vi "Controller Test Bench (14).vi"() -> ()   [LabVIEW 2022 SP3]
uses:
  WhiteNoise.ctl
  <vilib>/addons/System Identification/Model Typedefs.llb/si_generic model.ctl
  <vilib>/addons/System Identification/Model Typedefs.llb/SI Model Type.ctl
  <vilib>/addons/System Identification/Model Typedefs.llb/si_variables.ctl
  <vilib>/sound2/lvsound2.llb/Sound Data Format.ctl
  <vilib>/Utility/error.llb/DialogType.ctl
  <vilib>/sound2/lvsound2.llb/Sampling Mode.ctl
  <vilib>/Platform/TimedLoop/XDataNode/timing_clust.ctl
  <vilib>/Platform/TimedLoop/XDataNode/nitl_modes.ctl
  <vilib>/Platform/TimedLoop/XDataNode/wakeup.ctl
  <vilib>/Analysis/4window.llb/windowTd.ctl
  <vilib>/sound2/lvsound2.llb/Sound Output Task ID.ctl
  <vilib>/DAQmx/write.llb/DAQmx Write (Analog Wfm 1Chan NSamp).vi
  <vilib>/DAQmx/read.llb/DAQmx Read (Analog 1D Wfm NChan NSamp).vi
  <vilib>/DAQmx/create/channels.llb/DAQmx Create Channel (AI-Acceleration-Accelerometer).vi
  <vilib>/DAQmx/create/channels.llb/DAQmx Create Channel (AO-Voltage-Basic).vi
  <vilib>/DAQmx/configure/timing.llb/DAQmx Timing (Sample Clock).vi
  <vilib>/Platform/TimedLoop/scheduler/LVUserAPI/_suppVIs/Create_1kHz_TSource.vi
  <vilib>/DAQmx/miscellaneous.llb/DAQmx Fill In Error Info.vi
  <vilib>/DAQmx/configure/task.llb/DAQmx Configure Logging (TDMS).vi
  <vilib>/measure/maspectr.llb/FFT Spectrum (Mag-Phase) for N Chan.vi
  <vilib>/sound2/lvsound2.llb/Sound Output Set Volume (Single).vi
  <vilib>/sound2/lvsound2.llb/Sound Output Write (DBL).vi
  <vilib>/addons/control/pid/pid.llb/PID (DBL Array).vi
  <vilib>/sound2/lvsound2.llb/Sound Output Write (DBL Single).vi
  <vilib>/addons/System Identification/Data Preprocess.llb/SI Lowpass Filter (SISO Waveform).vi
  <vilib>/addons/System Identification/Parametric Estimation.llb/SI Estimate Discrete Transfer Function Model (Joint SISO Waveform).vi
  <vilib>/platform/TimedLoop/XDataNode/XDataNode.xnode
  <vilib>/measure/NI_MAPro.lvlib
  <resource>/objmgr/daqmx.rc
  <vilib>/Analysis/NI_AALPro.lvlib
  <vilib>/measure/NI_MABase.lvlib
  <vilib>/Platform/TimedLoop/XDataNode/XDNodeRunTimeDep.lvlib
  <vilib>/addons/control/pid/NI_PID_pid.lvlib
  <vilib>/addons/System Identification/NI_SysID.lvlib
panel:
  out "system model out":T1={"attributes"={"version"="1.0", "model type"=0, "input names"=[], "output names"=[], "notes"=""}, "coefficients"={"A "=[], "B"=[], "F"=[], "C"=[], "D"=[]}, "std deviations"={"A "=[], "B"=[], "F"=[], "C"=[], "D"=[]}, "coefficients covariance"=[], "noise variance"=[], "fs"=0.0, "system info"={"number of inputs"=0, "number of outputs"=0, "A order"=[], "B order"=[], "F order"=[], "C order"=[], "D order"=[], "Delays"=[]}, "kalman gain"=[], "initial state"=[], "trans func"=[], "zeros-poles"=[], "std of trans func"=[], "std of zeros-poles"=[], "trans func (noise)"=[], "std of trans func (noise)"=[], "zeros-poles (noise)"=[], "std of zeros-poles (noise)"=[], "Symbolic State Space Model"={"Symbolic A"=[], "Symbolic B"=[], "Symbolic C"=[], "Symbolic D"=[], "Symbolic K"=[], "Symbolic Initial State"=[]}, "delay"=[], "variables"=[], "grey trans func spec"={"orders of TF model"={" num order"=1, "den order"=2}, "# of zeros/poles at origin"={"zeros/poles"=1, "number "=0}, "delay initial?"=FALSE, "gain initial?"=FALSE}} {"grey trans func spec"."# of zeros/poles at origin"."zeros/poles" items=["zeros", "poles"]; "std of zeros-poles (noise)"."gain" format="%.2f"; "std of zeros-poles (noise)"."poles" format="%.2f"; "std of zeros-poles (noise)"."zeros" format="%.2f"; "zeros-poles (noise)"."gain" format="%.2f"; "zeros-poles (noise)"."poles" format="%.2f"; "zeros-poles (noise)"."zeros" format="%.2f"; "std of trans func (noise)"."alphas" format="%.2f"; "std of trans func (noise)"."betas" format="%.2f"; "trans func (noise)"."alphas" format="%.2f"; "trans func (noise)"."betas" format="%.2f"; "std of zeros-poles"."gain" format="%.2f"; "std of zeros-poles"."poles" format="%.2f"; "std of zeros-poles"."zeros" format="%.2f"; "std of trans func"."alphas" format="%.2f"; "std of trans func"."betas" format="%.2f"; "zeros-poles"."gain" format="%.2f"; "zeros-poles"."poles" format="%.2f"; "zeros-poles"."zeros" format="%.2f"; "trans func"."alphas" format="%.2f"; "trans func"."betas" format="%.2f"; "fs" format="%.2f"; "std deviations"."A" format="%.2f"; "std deviations"."D" format="%.2f"; "std deviations"."C" format="%.2f"; "std deviations"."F" format="%.2f"; "std deviations"."B" format="%.2f"; "coefficients"."A" format="%.2f"; "coefficients"."D" format="%.2f"; "coefficients"."C" format="%.2f"; "coefficients"."F" format="%.2f"; "coefficients"."B" format="%.2f"; "attributes"."model type" items=["Undefined", "AR", "ARX (SISO)", "ARX (MISO)", "ARX (MIMO)", "ARMAX (SISO)", "ARMAX (MISO)", "Output-Error (SISO)", "Output-Error (MISO)", "Box-Jenkins (SISO)", "Box-Jenkins (MISO)", "General Linear (SISO)", "General Linear (MISO)", "State-Space (SISO)", "State-Space (MISO)", "State-Space (MIMO)", "Transfer Function (SISO)", "Transfer Function (MISO)", "Transfer Function (MIMO)", "Zero-Pole-Gain (SISO)", "Zero-Pole-Gain (MISO)", "Zero-Pole-Gain (MIMO)"]}
  out "model coefficients":T4
  out "noise":dbl[](array[numeric])
  in  "Sample Rate":dbl=16384.0
  in  "TimeOut":dbl=30.0 format="%#_13g"
  in  "Cluster":T6={"Seed"=0.0, "Standard Deviation"=0.2, "Reset"=FALSE, "Iterator"=1.0, "Seed"=-1, "Stop 4"=FALSE} {"Standard Deviation" min=0.001 max=0.3 format="%0.2p"}
  out "ResponseLowPass":waveform(dbl)(graph)
  out "Output Signal 2":dbl[](graph)
  out "Timeout In(s)":i32 caption="Elapsed Time (s)" format="%.2f"
  in  "Acquisition\nPeriod(ms)":dbl=41.2
  out "Accel.1":waveform(dbl)(graph)
  in  "Active Control":bool
  in  "Tab Control":T7(tab)
  out "dt out (s)":dbl format="%.3f"
  in  "setpoint":dbl[](array[numeric])=[0.0] format="%.2f"
  in  "PID gains":T8(array[cluster])=[{"proportional gain (Kc)"=1.0, "integral time (Ti, min)"=0.01, "derivative time (Td, min)"=0.0}] {"derivative time (Td, min)" format="%.3f"; "integral time (Ti, min)" format="%.3f"; "proportional gain (Kc)" format="%.3f"}
  in  "dt (s)":dbl=-1.0 format="%.3f"
  in  "output range":cluster{"output high":dbl, "output low":dbl}[](array[cluster])=[{"output high"=100.0, "output low"=-100.0}] {"output low" format="%.2f"; "output high" format="%.2f"}
  in  "Upper Cut-Off":dbl=400.0
  in  "Lower Cut-Off":dbl=100.0
  in  "Setpoint":dbl
  in  "Gain":dbl min=0.0 step=0.01
  out "Output Signal":dynamicdata(graph)
  in  "Upper Cut-Off":dbl=400.0
  in  "Lower Cut-Off":dbl=100.0
  out "coefficients of transfer function model 2":cluster{"numerator":dbl[], "denominator":dbl[]}
  out "Accel.2":waveform(dbl)(graph)
  in  "Log Raw Data":bool
  out "Phase 2":cluster{"f0":dbl, "df":dbl, "phase":dbl[]}[](graph)
  out "Mag 2":cluster{"f0":dbl, "df":dbl, "magnitude":dbl[]}[](graph)
  in  "Show FFT":bool=TRUE
  in  "Log FFT":bool
  in  "Start Reading":bool=TRUE
  in  "Stop":bool
  # "Main\nSwitch"
  # "Active Controller"
  # "Output Noise"
  # "Output Amplitude"
  # "RAW - Accel. 1"
  # "Data Acquisition"
  # "FFT - Amplitude"
  # "FFT - Phase"
  # "RAW - Accel. 2"
  # "Runtime"
  # "Filter"
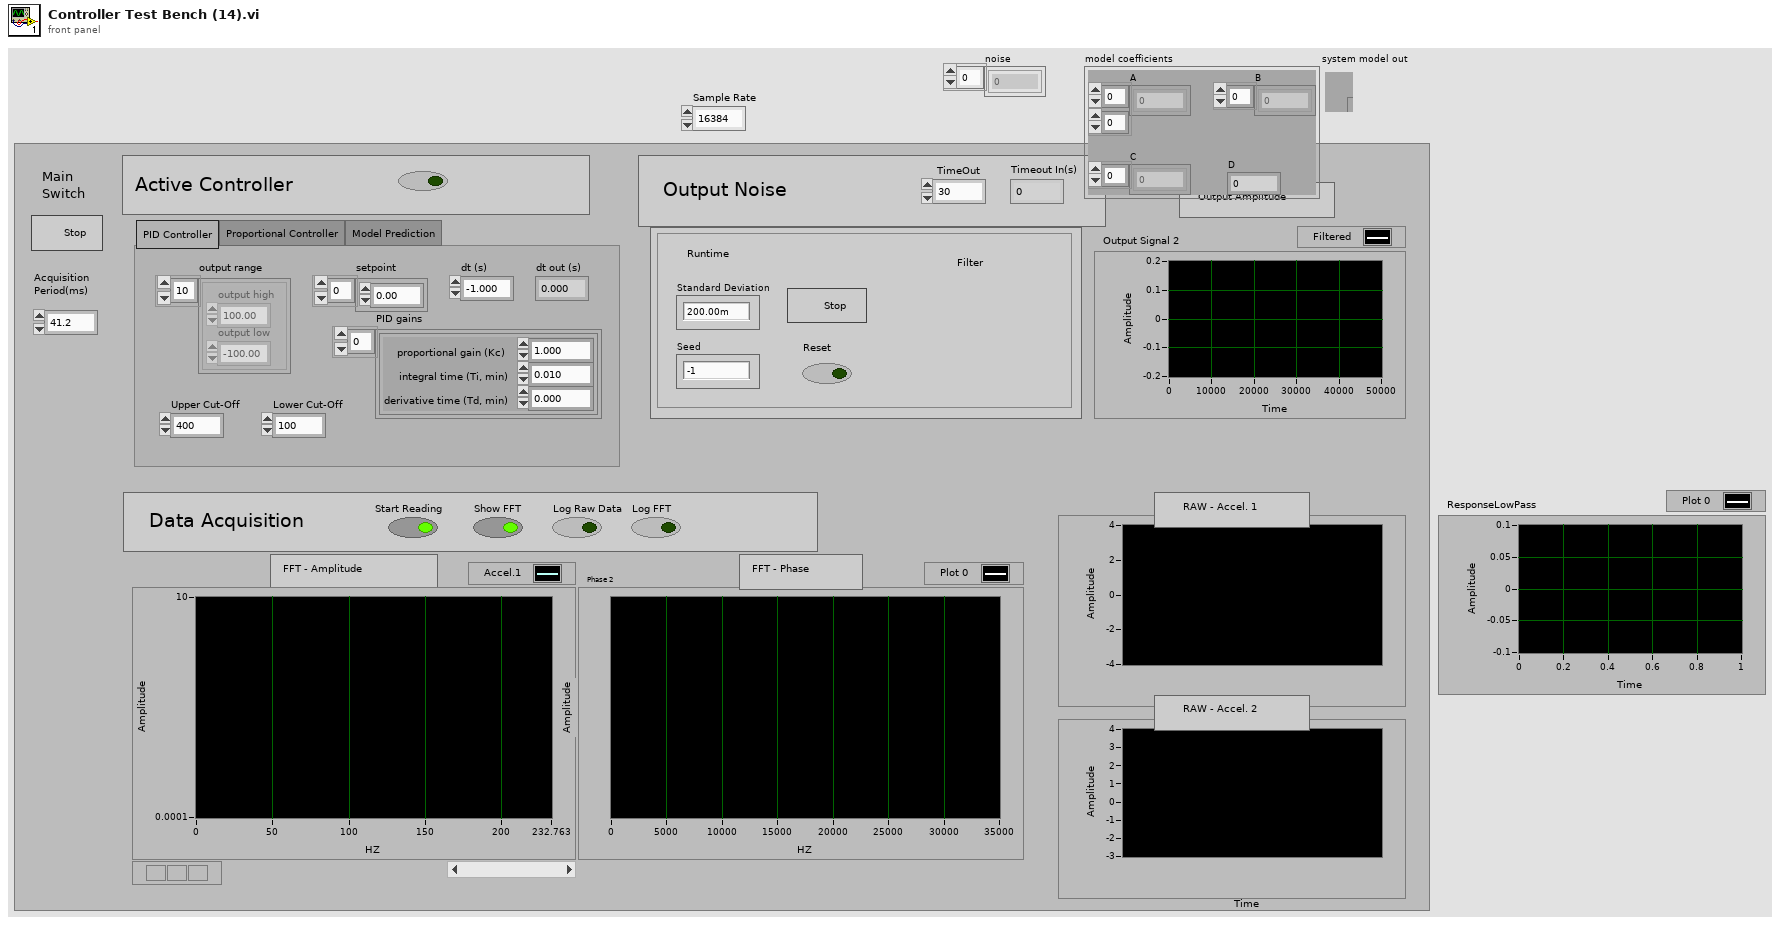
[diagram p1: front panel]
types:
  T1 = typedef "NI_SysID.lvlib/si_generic model.ctl" = cluster{"attributes":cluster{"version":string, "model type":T2, "input names":string[], "output names":string[], "notes":string}, "coefficients":cluster{"A ":dbl[][][], "B":dbl[][][], "F":dbl[][][], "C":dbl[][][], "D":dbl[][][]}, "std deviations":cluster{"A ":dbl[][][], "B":dbl[][][], "F":dbl[][][], "C":dbl[][][], "D":dbl[][][]}, "coefficients covariance":dbl[][][], "noise variance":dbl[][], "fs":dbl, "system info":cluster{"number of inputs":i32, "number of outputs":i32, "A order":i32[][], "B order":i32[][], "F order":i32[][], "C order":i32[][], "D order":i32[][], "Delays":i32[][]}, "kalman gain":dbl[][], "initial state":dbl[], "trans func":cluster{"betas":dbl[], "alphas":dbl[]}[][], "zeros-poles":cluster{"zeros":cdb[], "poles":cdb[], "gain":dbl}[][], "std of trans func":cluster{"betas":dbl[], "alphas":dbl[]}[][], "std of zeros-poles":cluster{"zeros":cdb[], "poles":cdb[], "gain":dbl}[][], "trans func (noise)":cluster{"betas":dbl[], "alphas":dbl[]}[][], "std of trans func (noise)":cluster{"betas":dbl[], "alphas":dbl[]}[][], "zeros-poles (noise)":cluster{"zeros":cdb[], "poles":cdb[], "gain":dbl}[][], "std of zeros-poles (noise)":cluster{"zeros":cdb[], "poles":cdb[], "gain":dbl}[][], "Symbolic State Space Model":cluster{"Symbolic A":string[][], "Symbolic B":string[][], "Symbolic C":string[][], "Symbolic D":string[][], "Symbolic K":string[][], "Symbolic Initial State":string[]}, "delay":dbl[][], "variables":T3, "grey trans func spec":cluster{"orders of TF model":cluster{" num order":i32, "den order":i32}, "# of zeros/poles at origin":cluster{"zeros/poles":u16, "number ":i32}, "delay initial?":bool, "gain initial?":bool}}
  T2 = typedef "NI_SysID.lvlib/SI Model Type.ctl" = u16
  T3 = typedef "NI_SysID.lvlib/si_variables.ctl" = cluster{"name":string, "initial guess":dbl, "upper limit":dbl, "lower limit":dbl, "value":dbl}[]
  T4 = cluster{"A":dbl[][], "B":dbl[], "C":dbl[], "D":dbl}
  T5 = typedef "WhiteNoise.ctl" = dbl
  T6 = cluster{"Seed":T5, "Standard Deviation":dbl, "Reset":bool, "Iterator":dbl, "Seed":i8, "Stop 4":bool}
  T7 = enum32{"PID Controller", "Proportional Controller", "Model Prediction"}
  T8 = cluster{"proportional gain (Kc)":dbl, "integral time (Ti, min)":dbl, "derivative time (Td, min)":dbl}[]
  T9 = typedef "Sampling Mode.ctl" = i32
  T10 = typedef "DialogType.ctl" = u16
  T11 = typedef "Sound Data Format.ctl" = cluster{"sample rate (S/s)":dbl, "number of channels":i32, "bits per sample":i32}
  T12 = typedef "Sound Output Task ID.ctl" = u32
  T13 = typedef "XDNodeRunTimeDep.lvlib/timing_clust.ctl" = cluster{"Expected End [f-1]":u64, "Actual End [f-1]":u64, "Finished Late? [f-1]":bool, "Expected End [i-1]":u64, "Actual End [i-1]":u64, "Finished Late? [i-1]":bool, "Expected Start [i]":u64, "Actual Start [i]":u64, "Expected Start [f]":u64, "Actual Start [f]":u64, "Source Name":string, "Structure Name":string, "Period":i64, "Deadline":i64, "Offset":i64, "Start":i64, "Priority":i32, "Timeout":i32, "Mode":T14, "Wakeup Reason":T15, "Error":errorcluster, "Source Type":string, "Secondary Source Type":string, "Global End Time":u64, "Global Start Time":u64, "Frame Duration":u64, "Iteration Duration":u64, "Assigned CPU":i32, "I/O Scan Engine Mode":u32}
  T14 = typedef "XDNodeRunTimeDep.lvlib/nitl_modes.ctl" = enum32{"No Change", "Process missed periods, maintain original phase", "Discard missed periods, maintain original phase", "Process missed periods, ignore original phase", "Discard missed periods, ignore original phase"}
  T15 = typedef "XDNodeRunTimeDep.lvlib/wakeup.ctl" = enum32{"Normal", "Aborted", "Asynchronous wakeup", "Timing source error", "Timed loop error", "Timeout"}
  T16 = typedef "NI_AALPro.lvlib/windowTd.ctl" = u32
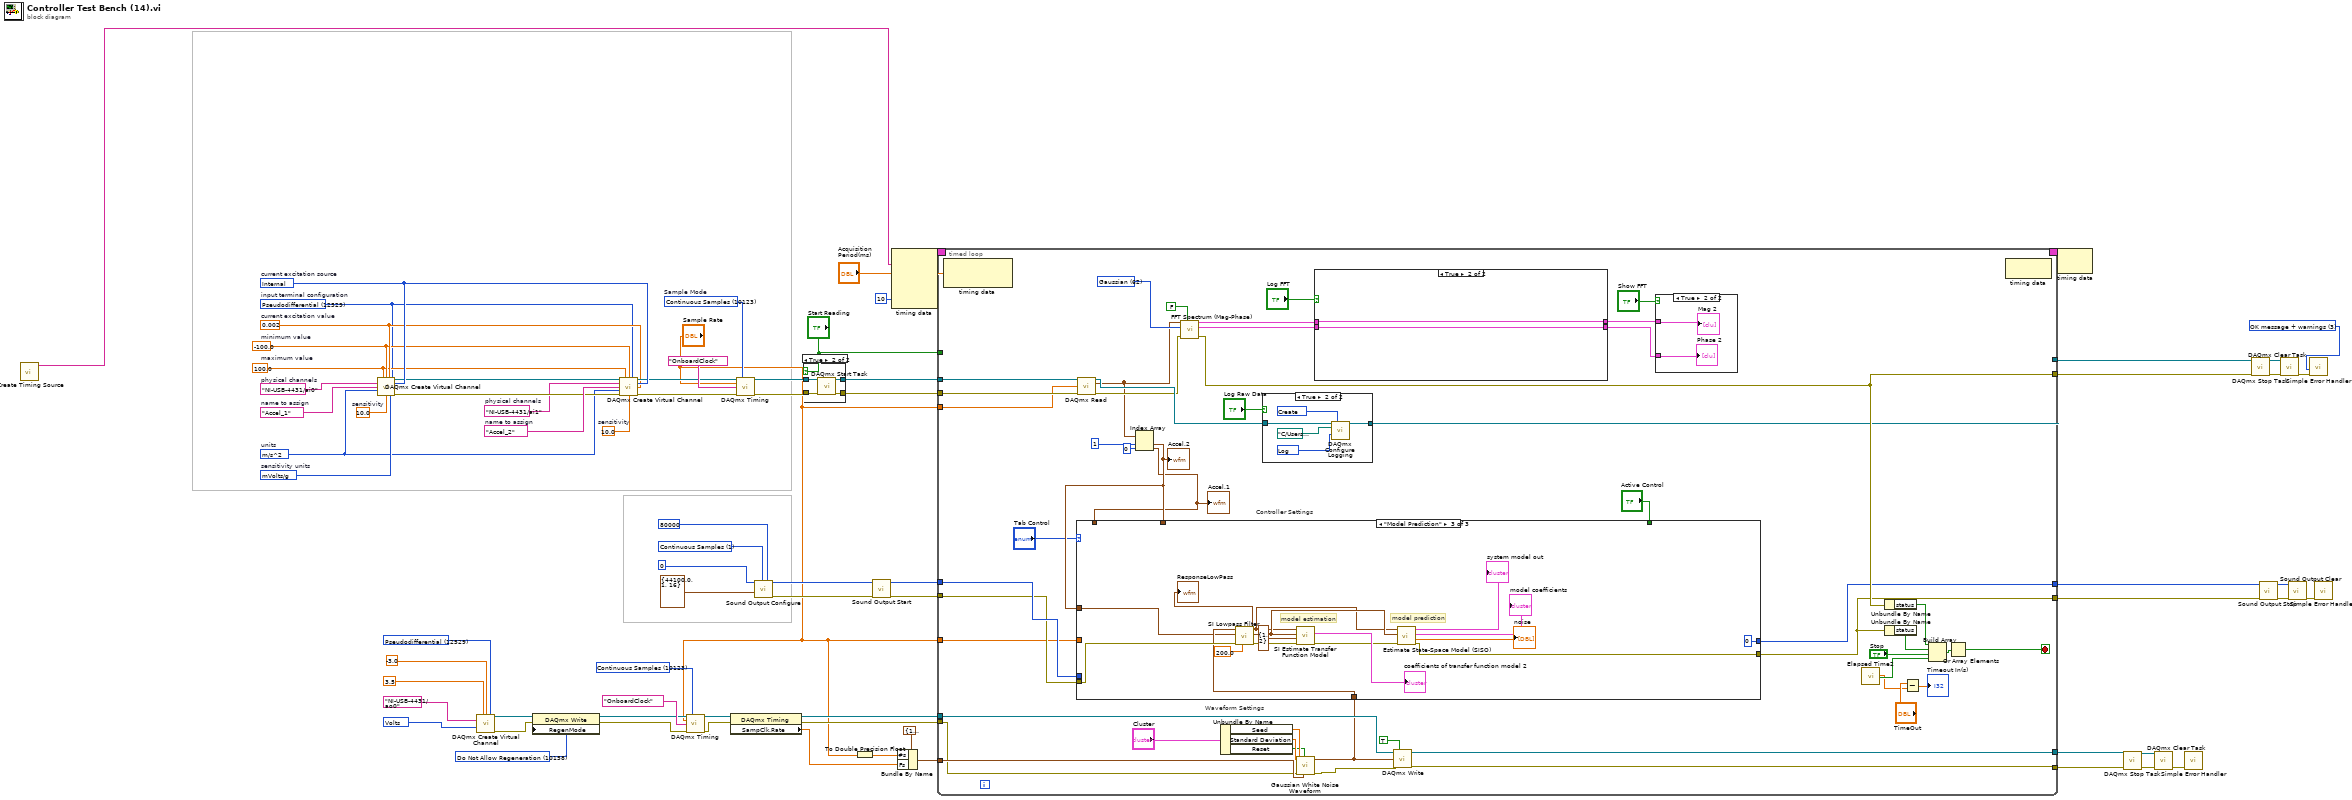
[diagram p0: block diagram]
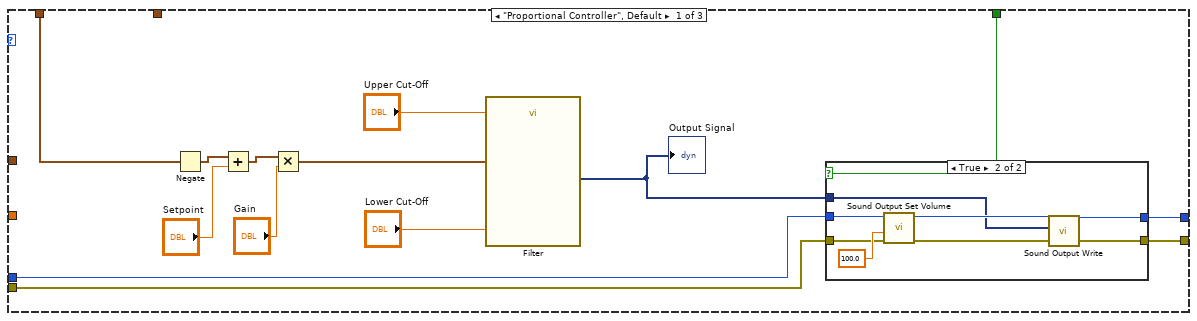
[diagram p2: hidden frame]
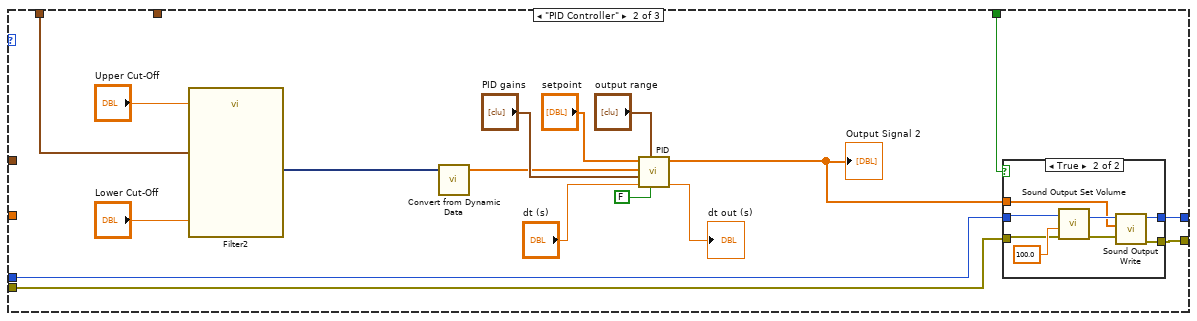
[diagram p4: hidden frame]
diagram:
  w15 = 10123 items=["Finite Samples"=10178, "Continuous Samples"=10123, "Hardware Timed Single Point"=12522] ("sample mode")
  w19 = 10158 items=["Allow Regeneration"=10097, "Do Not Allow Regeneration"=10158] ("RegenMode")
  w24 = 12529 items=["Default"=-1, "RSE"=10083, "Differential"=10106, "Pseudodifferential"=12529] ("output terminal configuration")
  w22 = 10348 items=["Volts"=10348, "From Custom Scale"=10065] ("units")
  w62 = 12509 items=["mVolts/g"=12509, "Volts/g"=12510]  # sensitivity units
  w63 = 10.0  # sensitivity
  w54 = 0.002  # current excitation value
  w57 = 10200 items=["Internal"=10200, "External"=10167, "None"=10230]  # current excitation source
  w47 = tag "NI-USB-4431/ai0"  # physical channels
  w61 = 10123 items=["Finite Samples"=10178, "Continuous Samples"=10123, "Hardware Timed Single Point"=12522]  # Sample Mode
  w50 = 12529 items=["default"=-1, "RSE"=10083, "NRSE"=10078, "Differential"=10106, "Pseudodifferential"=12529]  # input terminal configuration
  w53 = -100.0  # minimum value
  w52 = 100.0  # maximum value
  w64 = "Accel_1"  # name to assign
  w51 = 12470 items=["g"=10186, "m/s^2"=12470, "in/s^2"=12471, "From Custom Scale"=10065]  # units
  w65 = 10.0  # sensitivity
  w48 = tag "NI-USB-4431/ai1"  # physical channels
  w59 = "Accel_2"  # name to assign
  w66 = T9 1 items=["Finite Samples", "Continuous Samples"] ("sample mode")
  w67 = T10 3 items=["no dialog", "OK message", "continue or stop message", "OK message + warnings", "continue/stop + warnings"] ("type of dialog (OK msg:1)")
  n1 = call-poly <vilib>:"Create Timing Source.vi"() -> ("name (out)"=w27:string)  [unwired: 10 in, 1 out]
  n2 = call-poly <vilib>:"DAQmx Create Virtual Channel.vi"("maximum value"=w52, "minimum value"=w53, "input terminal configuration"=w50, "physical channels"=w47, "current excitation source"=w57, "name to assign"=w64, "current excitation value"=w54, "units"=w51, "sensitivity"=w63, "sensitivity units"=w62) -> ("task out"=w49:refnum<k21>, "error out"=w58:errorcluster)  [unwired: 4 in]
  n3 = call-poly <vilib>:"DAQmx Create Virtual Channel.vi"("maximum value"=3.5, "minimum value"=-3.0, "output terminal configuration"=w24, "physical channels"=tag "NI-USB-4431/ao0", "units"=w22) -> ("task out"=w18:refnum<k21>, "error out"=w20:errorcluster)  [unwired: 9 in]
  n4 = property class="DAQmx Write"(reference=w18, error in=w20, "RegenMode"=w19) -> (reference out=w16:refnum<k21>, error out=w17:errorcluster)
  n5 = call-poly <vilib>:"DAQmx Create Virtual Channel.vi"("task in"=w49, "maximum value"=w52, "minimum value"=w53, "input terminal configuration"=w50, "physical channels"=w48, "current excitation source"=w57, "name to assign"=w59, "current excitation value"=w54, "units"=w51, "error in"=w58, "sensitivity"=w65) -> ("task out"=w56:refnum<k21>, "error out"=w55:errorcluster)  [unwired: 3 in]
  n6 = call-poly <vilib>:"DAQmx Timing.vi"("task/channels in"=w16, "sample mode"=w15, "rate"="Sample Rate", "source"=tag "OnboardClock" ("Sample Clock Source"), "error in"=w17) -> ("task out"=w11:refnum<k21>, "error out"=w10:errorcluster)  [unwired: 9 in]
  n7 = property class="DAQmx Timing"(reference=w11, error in=w10) -> (reference out=w8:refnum<k21>, error out=w7:errorcluster, "SampClk.Rate"=w12:dbl)
  n8 = call-poly <vilib>:"DAQmx Timing.vi"("task/channels in"=w56, "sample mode"=w61, "rate"="Sample Rate", "source"=tag "OnboardClock" ("Sample Clock Source"), "error in"=w55) -> ("task out"=w45:refnum<k21>, "error out"=w46:errorcluster)  [unwired: 9 in]
  n9 = call <vilib>:"Sound Output Configure.vi"("number of samples/ch"=80000 ("Number of Samples/ch"), "sample mode"=w66, "sound format"=T11 {"sample rate (S/s)"=44100.0, "number of channels"=1, "bits per sample"=16} ("Sound Format"), "device ID"=u32 0 ("Device ID")) -> ("error out"=w41:errorcluster, "task ID"=w40:T12)  [unwired: 6 in]
  n10 = case shown="True" "Start Reading" {
    tunnel: w46 -> [w75 w80]
    tunnel: w45 -> [w76 w79]
    tunnel: [w76 w78] -> w33
    tunnel: [w75 w77] -> w34
    frame False {
    }
    frame True {
      n11 = call <vilib>:"DAQmx Start Task.vi"("task/channels in"=w79, "error in"=w80) -> ("task out"=w78:refnum<k21>, "error out"=w77:errorcluster)  [unwired: 12 in]
    }
  }
  n12 = To Double Precision Float(number="Sample Rate") -> (double precision float=w13:dbl)
  n13 = call <vilib>:"Sound Output Start.vi"("error in (no error)"=w41, "task ID"=w40) -> ("error out"=w35:errorcluster, "task ID out"=w36:T12)  [unwired: 8 in]
  n14 = node-c288(w27, "Acquisition\nPeriod(ms)", i64 10 ("Offset")) -> (w39:T13)  [unwired: 2 in]
  n15 = Bundle By Name(cluster=cluster{"Fs":dbl, "#s":dbl} {"Fs"=1000.0, "#s"=1000.0} ("sampling info"), "#s"=w13, "Fs"=w12) -> (w9:cluster{"Fs":dbl, "#s":dbl})
  n16 = timed-loop {
    timing: w39 -> [_]
    timing-out: [_] -> w38
    tunnel: "Start Reading" -> [_]
    tunnel: w36 -> [w129]
    tunnel: w35 -> [w128]
    tunnel: w34 -> [w127]
    tunnel: w33 -> [w126]
    tunnel: [w125] -> w32
    tunnel: [w124] -> w31
    tunnel: [w123] -> w30
    tunnel: [w122] -> w29
    tunnel: w9 -> [w118]
    tunnel: w8 -> [w117]
    tunnel: w7 -> [w116]
    tunnel: "Sample Rate" -> [w86]
    tunnel: [w85] -> w3
    tunnel: [w84] -> w2
    tunnel: "Sample Rate" -> [w83]
    stop <- w121 stop-if-true
    w101 = T16 62 items=["Rectangle"=0, "Hanning"=1, "Hamming"=2, "Blackman-Harris"=3, "Exact Blackman"=4, "Blackman"=5, "Flat Top"=6, "4 Term B-Harris "=7, "7 Term B-Harris"=8, "Low Sidelobe"=9, "Blackman Nuttall"=11, "Triangle"=30, "Bartlett-Hanning"=31, "Bohman"=32, "Parzen"=33, "Welch"=34, "Kaiser"=60, "Dolph-Chebyshev"=61, "Gaussian"=62] ("window")
    # "Controller Settings"
    # "Waveform Settings"
    n17 = node-c288() -> ()  [unwired: 1 in, 2 out]
    n18 = call-poly <vilib>:"DAQmx Read.vi"("task/channels in"=w126, "number of samples per channel"=w83, "error in"=w127) -> ("task out"=w113:refnum<k21>, "data"=w96:waveform(dbl)[], "error out"=w102:errorcluster)  [unwired: 10 in]
    n19 = Index Array(array=w96, index #1=1 ("index"), index #2=0 ("index")) -> (element #1=w115:waveform(dbl), element #2=w81:waveform(dbl))
    "Accel.2" <- w115
    "Accel.1" <- w81
    n20 = call-poly <vilib>:"FFT Spectrum (Mag-Phase).vi"("restart averaging (F)"=FALSE, "error in (no error)"=w102, "window"=w101, "time signals"=w96) -> ("error out"=w125:errorcluster, "phases"=w107:cluster{"f0":dbl, "df":dbl, "phase":dbl[]}[], "magnitudes"=w108:cluster{"f0":dbl, "df":dbl, "magnitude":dbl[]}[])  [unwired: 3 in, 2 out]
    n21 = Unbundle By Name("Cluster") -> ("Seed"=w90:T5, "Standard Deviation"=w89:dbl, "Reset"=w88:bool)
    n22 = case shown="True" "Log Raw Data" {
      tunnel: w113 -> [w202 w204]
      tunnel: [w202 w203] -> w124
      frame False {
      }
      frame True {
        w205 = 15848 items=["Open"=10437, "Open or Create"=15846, "Create or Replace"=15847, "Create"=15848] ("operation")
        w206 = 15844 items=["Off"=10231, "Log"=15844, "Log and Read"=15842] ("logging mode")
        n23 = call-poly <vilib>:"DAQmx Configure Logging.vi"("task/channels in"=w204, "operation"=w205, "file path"=path "C:/Users/LAV-UFSC/Documents/LAV - TCC", "logging mode"=w206) -> ("task out"=w203:refnum<k21>)  [unwired: 10 in, 1 out]
      }
    }
    n24 = call <vilib>:"Gaussian White Noise Waveform.vi"("sampling info"=w118, "reset signal"=w88, "error in (no error)"=w116, "seed"=w90, "standard deviation"=w89) -> ("error out"=w119:errorcluster, "signal out"=w91:waveform(dbl))  [unwired: 5 in]
    n25 = case shown="\"Model Prediction\"" "Tab Control" {
      tunnel: w81 -> [w139 w154 _]
      tunnel: w129 -> [w135 w165 _]
      tunnel: w128 -> [w136 w164 w193]
      tunnel: "Active Control" -> [w134 w163 _]
      tunnel: [w138 w162 T12 0 ("task ID out")] -> w123
      tunnel: [w137 w161 w187] -> w122
      tunnel: w115 -> [_ _ _]
      tunnel: w115 -> [_ _ w188]
      tunnel: w91 -> [_ _ w189]
      tunnel: w86 -> [_ _ _]
      frame "Proportional Controller", Default {
        n26 = Negate(x=w139) -> (-x=w142:waveform(dbl))
        n27 = Add(x=w142, y="Setpoint") -> (x+y=w141:waveform(dbl))
        n28 = Multiply(x=w141, y="Gain") -> (x*y=w133:waveform(dbl))
        n29 = call "Filter"("Lower Cut-Off"="Lower Cut-Off", "Upper Cut-Off"="Upper Cut-Off", "Signal"=w133) -> ("Filtered Signal"=w132:dynamicdata)  [unwired: 7 in, 1 out]
        "Output Signal" <- w132
        n30 = case shown="True" w134 {
          tunnel: w136 -> [w145 w151]
          tunnel: [w145 w148] -> w137
          tunnel: w135 -> [w144 w152]
          tunnel: [w144 w147] -> w138
          tunnel: w132 -> [_ w146]
          frame False {
          }
          frame True {
            n31 = call-poly <vilib>:"Sound Output Set Volume.vi"("error in (no error)"=w151, "volume"=100.0, "task ID"=w152) -> ("error out"=w149:errorcluster, "task ID out"=w150:T12)  [unwired: 7 in]
            n32 = call-poly <vilib>:"Sound Output Write.vi"("error in (no error)"=w149, "data"=w146, "task ID"=w150) -> ("error out"=w148:errorcluster, "task ID out"=w147:T12)  [unwired: 7 in]
          }
        }
      }
      frame "PID Controller" {
        n33 = call "Filter2"("Lower Cut-Off"="Lower Cut-Off", "Upper Cut-Off"="Upper Cut-Off", "Signal"=w154) -> ("Filtered Signal"=w156:dynamicdata)  [unwired: 7 in, 1 out]
        n34 = call "Convert from Dynamic Data"("Dynamic Data Type"=w156) -> ("Array"=w155:dbl[])  [unwired: 3 in]
        n35 = call-poly <vilib>:"PID.vi"("reinitialize? (F)"=FALSE, "output range"="output range", "dt (s)"="dt (s)", "PID gains"="PID gains", "process variable"=w155, "setpoint"="setpoint") -> ("dt out (s)"=→"dt out (s)":dbl, "output"=w157:dbl[])  [unwired: 4 in]
        "Output Signal 2" <- w157
        n36 = case shown="True" w163 {
          tunnel: w164 -> [w172 w178]
          tunnel: [w172 w175] -> w161
          tunnel: w165 -> [w171 w179]
          tunnel: [w171 w174] -> w162
          tunnel: w157 -> [_ w173]
          frame False {
          }
          frame True {
            n37 = call-poly <vilib>:"Sound Output Set Volume.vi"("error in (no error)"=w178, "volume"=100.0, "task ID"=w179) -> ("error out"=w176:errorcluster, "task ID out"=w177:T12)  [unwired: 7 in]
            n38 = call-poly <vilib>:"Sound Output Write.vi"("error in (no error)"=w176, "data"=w173, "task ID"=w177) -> ("error out"=w175:errorcluster, "task ID out"=w174:T12)  [unwired: 7 in]
          }
        }
      }
      frame "Model Prediction" {
        # "model prediction"
        # "model estimation"
        n39 = call-poly <vilib>:"SI Lowpass Filter.vi"("cutoff frequency"=200.0, "error in (no error)"=w193, "response signal in"=w188, "stimulus signal in"=w189) -> ("error out"=w194:errorcluster, "response signal out"=w185:waveform(dbl), "stimulus signal out"=w184:waveform(dbl))  [unwired: 5 in]
        "ResponseLowPass" <- w184
        n40 = call-poly <vilib>:"SI Estimate Transfer Function Model.vi"("error in (no error)"=w194, "orders of transfer function model"=cluster{" num order":i32, "den order":i32} {" num order"=1, "den order"=2}, "response signal"=w185, "stimulus signal"=w184) -> ("error out"=w186:errorcluster, "coefficients of transfer function model"=→"coefficients of transfer function model 2":cluster{"numerator":dbl[], "denominator":dbl[]})  [unwired: 5 in, 1 out]
        n41 = call "Estimate State-Space Model (SISO)"("error in (no error)"=w186, "response signal"=w185, "stimulus signal"=w184) -> ("error out"=w187:errorcluster, "noise"=→"noise":dbl[], "model coefficients"=→"model coefficients":T4, "system model out"=→"system model out":T1)  [unwired: 5 in]
      }
    }
    n42 = case shown="True" "Log FFT" {
      tunnel: w108 -> [w196 w199]
      tunnel: w107 -> [w197 w198]
      tunnel: [w197 w198] -> w106
      tunnel: [w196 w199] -> w105
      frame False {
      }
      frame True {
      }
    }
    n43 = call-poly <vilib>:"DAQmx Write.vi"("task/channels in"=w117, "auto start"=TRUE, "data"=w91, "error in"=w119) -> ("task out"=w84:refnum<k21>, "error out"=w85:errorcluster)  [unwired: 9 in, 1 out]
    n44 = case shown="True" "Show FFT" {
      tunnel: w105 -> [_ w201]
      tunnel: w106 -> [_ w200]
      frame False {
      }
      frame True {
        "Mag 2" <- w201
        "Phase 2" <- w200
      }
    }
    n45 = call "Elapsed Time2"() -> ("Elapsed Time (s)"=w92:dbl, "Time has Elapsed"=w95:bool)  [unwired: 12 in, 6 out]
    n46 = Unbundle By Name(w125) -> ("status"=w100:bool)
    n47 = Unbundle By Name(w122) -> ("status"=w104:bool)
    n48 = Subtract(x="TimeOut", y=w92) -> (x-y=→"Timeout In(s)":dbl)
    n49 = Build Array(w100, w104, "Stop", w95) -> (w111:bool[])
    n50 = Or Array Elements(Boolean array=w111) -> (logical OR=w121:bool)
    n51 = node-c288() -> ()  [unwired: 1 in, 1 out]
  }
  n52 = node-c288(w38) -> ()  [unwired: 1 out]
  n53 = call <vilib>:"DAQmx Stop Task.vi"("task/channels in"=w2, "error in"=w3) -> ("task out"=w6:refnum<k21>, "error out"=w5:errorcluster)  [unwired: 12 in]
  n54 = call <vilib>:"DAQmx Clear Task.vi"("task in"=w6, "error in"=w5) -> ("error out"=w4:errorcluster)  [unwired: 13 in]
  n55 = call <vilib>:"Simple Error Handler.vi"("error in (no error)"=w4) -> ()  [unwired: 4 in, 5 out]
  n56 = call <vilib>:"DAQmx Stop Task.vi"("task/channels in"=w31, "error in"=w32) -> ("task out"=w70:refnum<k21>, "error out"=w69:errorcluster)  [unwired: 12 in]
  n57 = call <vilib>:"Sound Output Stop.vi"("error in (no error)"=w29, "task ID"=w30) -> ("error out"=w44:errorcluster, "task ID out"=w43:T12)  [unwired: 8 in]
  n58 = call <vilib>:"DAQmx Clear Task.vi"("task in"=w70, "error in"=w69) -> ("error out"=w71:errorcluster)  [unwired: 13 in]
  n59 = call <vilib>:"Sound Output Clear.vi"("error in (no error)"=w44, "task ID"=w43) -> ("error out"=w42:errorcluster)  [unwired: 9 in]
  n60 = call <vilib>:"Simple Error Handler.vi"("type of dialog (OK msg:1)"=w67, "error in (no error)"=w71) -> ()  [unwired: 3 in, 5 out]
  n61 = call <vilib>:"Simple Error Handler.vi"("error in (no error)"=w42) -> ()  [unwired: 4 in, 5 out]
